vi "Configure Synthesizer Mode.vi"(8 "error in (no error)":errorcluster, 10 "Synthesizer Mode":enum16{"Normal", "Low Noise"}(ring), 11 "SigGen-SMBV in":refnum<class "VSG-SMBV.lvclass">) -> (0 "error out":errorcluster, 3 "SigGen-SMBV out":refnum<class "VSG-SMBV.lvclass">)   [LabVIEW 2020, in "VSG-SMBV.lvclass"]
uses:
  VSG-SMBV.lvclass
  Vector Signal Generator.lvclass
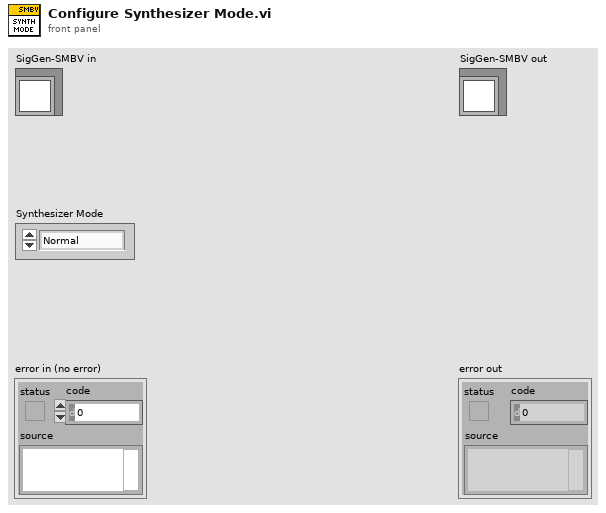
[diagram p1: front panel]
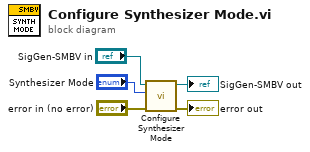
[diagram p0: block diagram]
diagram:
  n1 = call-parent "Configure Synthesizer Mode.vi"("error in (no error)"="error in (no error)", "Synthesizer Mode"="Synthesizer Mode", "Signal Generator in"="SigGen-SMBV in") -> ("error out"=→"error out":errorcluster, "Signal Generator out"=→"SigGen-SMBV out":refnum<class "VSG-SMBV.lvclass">)  [unwired: 7 in]
